vi "RS232.vi"() -> ()   [LabVIEW 2012]
uses:
  <vilib>/Instr/_visa.llb/VISA Configure Serial Port (Instr).vi
  Globalna_Variabla.vi
panel:
  out "Treshold 2":dbl
  in  "Tab Control":enum32{"Setings", "Recived Data"}(tab)
  out "Read Buffer":string
  in  "VISA resource name":refnum<visa-resource-name>="COM19"
  in  "Baud Rate (9600)":u32=115200
  in  "Reciving Byte Count (9)":u32=9
  in  "length":i32=100
  in  "index":i32
  out "Buffer Index":i8
  out "Iteration":i32
  out "Recived bytes (5)":string[](array[string])
  out "String Output (4)":string[](array[string])
  in  "Split Index (5)":i32=5
  out "index of NaN":i32
  out "Treshold":dbl
  out "size(s)":i32
  in  "Sekvenca":dbl[](array[numeric])
  out "Double Output (4)":dbl[](array[numeric])
  in  "stop":bool
  # "Brisanje Sekvence"
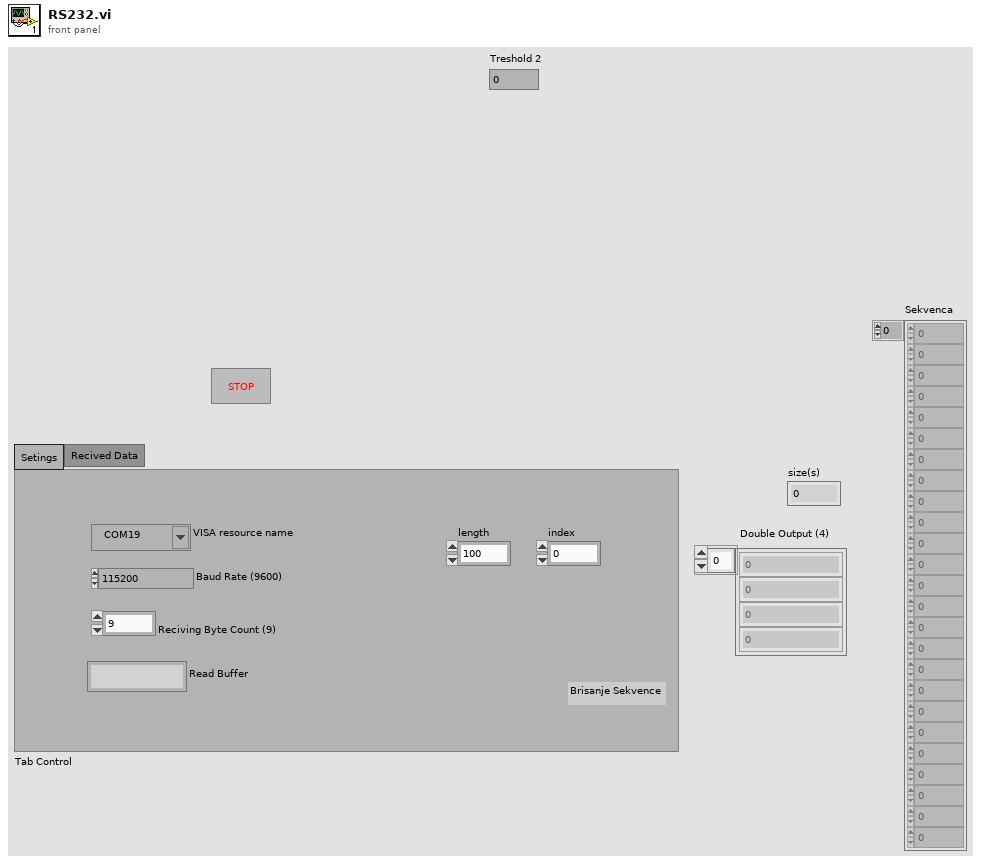
[diagram p1: front panel]
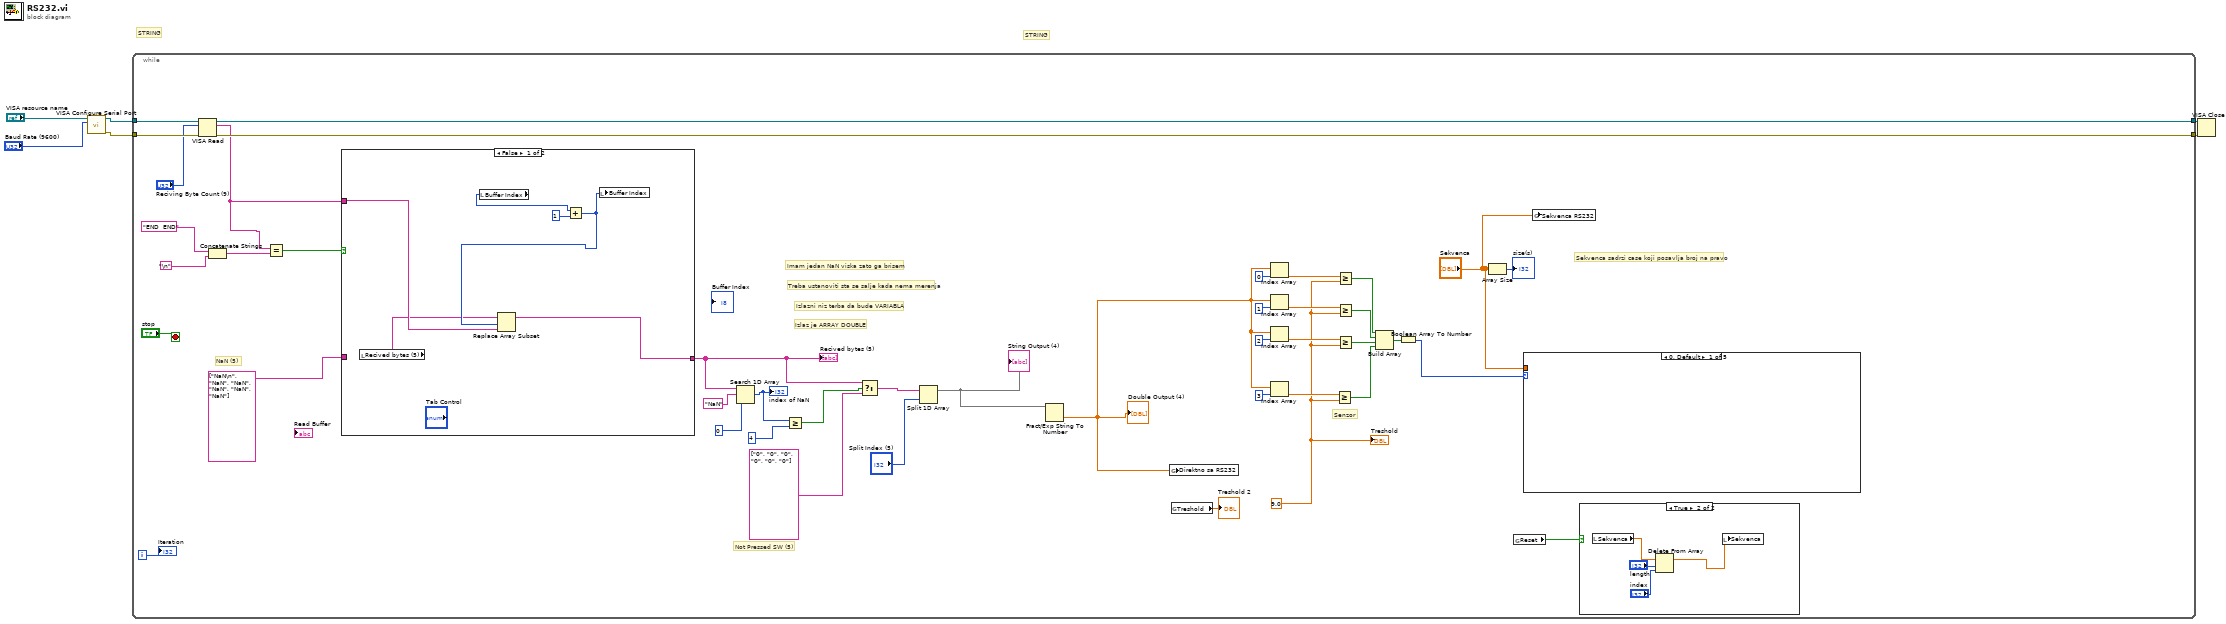
[diagram p0: block diagram]
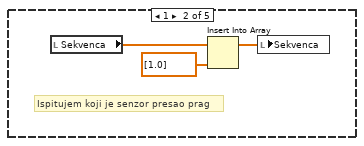
[diagram p3: hidden frame]
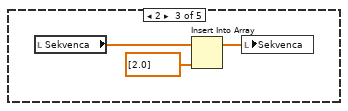
[diagram p4: hidden frame]
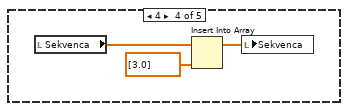
[diagram p5: hidden frame]
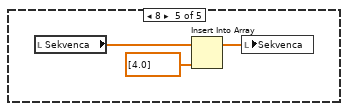
[diagram p6: hidden frame]
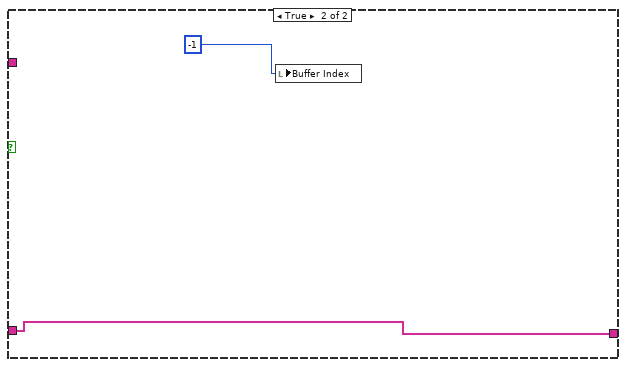
[diagram p7: hidden frame]
diagram:
  # "STRING"
  # "STRING"
  n1 = call-poly "VISA Configure Serial Port"("VISA resource name"="VISA resource name", "baud rate (9600)"="Baud Rate (9600)") -> ("VISA resource name out"=w5:refnum<visa-resource-name>, "error out"=w3:errorcluster)  [unwired: 12 in]
  n2 = while {
    tunnel: w5 -> [w48]
    tunnel: [w47] -> w4
    tunnel: w3 -> [w46]
    tunnel: [w45] -> w2
    i -> [w28]
    stop <- "stop" stop-if-true
    w8 = 9.0 ("y")
    # "Senzor"
    # "Sekvenca sadrzi case koji posavlja broj na pravo"
    # "Izlaz je ARRAY DOUBLE"
    # "Izlazni niz terba da bude VARIABLA"
    # "NaN (5)"
    # "Not Pressed SW (5)"
    # "Treba ustanoviti sta se salje kada nema merenja"
    # "Imam jedan NaN viska zato ga brisem"
    n3 = VISA Read(VISA resource name=w48, byte count="Reciving Byte Count (9)", error in (no error)=w46) -> (VISA resource name out=w47:refnum<visa-resource-name>, read buffer=w40:string, error out=w45:errorcluster)  [unwired: 1 out]
    n4 = Concatenate Strings("END  END" ("y"), "\n") -> (w43:string)
    n5 = Equal?(x=w40, y=w43) -> (x = y?=w33:bool)
    n6 = case shown="False" w33 {
      tunnel: w40 -> [w67 _]
      tunnel: [w71 w72] -> w36
      tunnel: string[] ["NaN\n", "NaN", "NaN", "NaN", "NaN", "NaN"] -> [_ w72]
      frame False {
        n7 = local read "Recived bytes (5)"() -> (w66:string[])
        n8 = local read "Buffer Index"() -> (w69:i8)
        n9 = Add(x=w69, y=i8 1) -> (x+y=w68:i8)
        n10 = Replace Array Subset(array=w66, new element=w67, index=w68) -> (w71:string[])
        n11 = local write "Buffer Index"(w68) -> ()
      }
      frame True {
        n12 = local write "Buffer Index"(i8 -1 ("Numeric")) -> ()
      }
    }
    "Recived bytes (5)" <- w36
    n13 = Search 1D Array(1D array=w36, element="NaN", start index (0)=0) -> (index of element=w37:i32)
    "index of NaN" <- w37
    n14 = Greater Or Equal?(x=w37, y=4) -> (x >= y?=w35:bool)
    n15 = Select(t=w36, s=w35, f=string[] ["0", "0", "0", "0", "0", "0"]) -> (s? t:f=w32:string[])
    n16 = Split 1D Array(array=w32, index="Split Index (5)") -> (first subarray=w27:string[])  [unwired: 1 out]
    "String Output (4)" <- w27
    n17 = Fract/Exp String To Number(string=w27) -> (number=w11:dbl[])  [unwired: 3 in, 1 out]
    "Double Output (4)" <- w11
    n18 = global write "Globalna_Variabla.vi" "Direktno sa RS232"(w11) -> ()
    n19 = global read "Globalna_Variabla.vi" "Treshold"() -> (→"Treshold 2":dbl)
    n20 = Index Array(array=w11, index=0) -> (element=w15:dbl)
    n21 = Index Array(array=w11, index=1) -> (element=w14:dbl)
    n22 = Index Array(array=w11, index=2) -> (element=w13:dbl)
    n23 = Index Array(array=w11, index=3) -> (element=w10:dbl)
    n24 = Greater Or Equal?(x=w10, y=w8) -> (x >= y?=w19:bool)
    n25 = Greater Or Equal?(x=w15, y=w8) -> (x >= y?=w22:bool)
    n26 = Greater Or Equal?(x=w14, y=w8) -> (x >= y?=w21:bool)
    n27 = Greater Or Equal?(x=w13, y=w8) -> (x >= y?=w20:bool)
    n28 = Build Array(w22, w21, w20, w19) -> (w18:bool[])
    n29 = Boolean Array To Number(Boolean array=w18) -> (number=w17:u32)
    n30 = Array Size(array="Sekvenca") -> (size(s)=→"size(s)":i32)
    n31 = global read "Globalna_Variabla.vi" "Reset"() -> (w7:bool)
    n32 = case shown="0, Default" w17 {
      tunnel: "Sekvenca" -> [_ _ _ _ _]
      frame 0, Default {
      }
      frame 1 {
        # "Ispitujem koji je senzor presao prag"
        n33 = local read "Sekvenca"() -> (w54:dbl[])
        n34 = Insert Into Array(array=w54, new element=dbl[] [1.0]) -> (w56:dbl[])  [unwired: 1 in]
        n35 = local write "Sekvenca"(w56) -> ()
      }
      frame 2 {
        n36 = local read "Sekvenca"() -> (w57:dbl[])
        n37 = Insert Into Array(array=w57, new element=dbl[] [2.0]) -> (w59:dbl[])  [unwired: 1 in]
        n38 = local write "Sekvenca"(w59) -> ()
      }
      frame 4 {
        n39 = local read "Sekvenca"() -> (w60:dbl[])
        n40 = Insert Into Array(array=w60, new element=dbl[] [3.0]) -> (w62:dbl[])  [unwired: 1 in]
        n41 = local write "Sekvenca"(w62) -> ()
      }
      frame 8 {
        n42 = local read "Sekvenca"() -> (w63:dbl[])
        n43 = Insert Into Array(array=w63, new element=dbl[] [4.0]) -> (w65:dbl[])  [unwired: 1 in]
        n44 = local write "Sekvenca"(w65) -> ()
      }
    }
    n45 = global write "Globalna_Variabla.vi" "Sekvenca RS232"("Sekvenca") -> ()
    n46 = case shown="True" w7 {
      frame False {
      }
      frame True {
        n47 = local read "Sekvenca"() -> (w52:dbl[])
        n48 = Delete From Array(array=w52, length="length", index="index") -> (array with subset deleted=w53:dbl[])  [unwired: 1 out]
        n49 = local write "Sekvenca"(w53) -> ()
      }
    }
    "Iteration" <- w28
    "Treshold" <- w8
  }
  n50 = VISA Close(VISA resource name=w4, error in (no error)=w2) -> ()  [unwired: 1 out]
